vi "Delete Entity.vi"(8 "error in (no error)":errorcluster, 9 "enqueuer":refnum<class "Message Enqueuer.lvclass">, 10 "entity type":i32, 11 "entity table in":refnum<class "Entity Table.lvclass">) -> (0 "error out":errorcluster, 3 "entity table out":refnum<class "Entity Table.lvclass">)   [LabVIEW 2020, in "Entity Table.lvclass"]
doc: "Delete an actor from the entity table."
uses:
  Entity Table.lvclass
  <vilib>/ActorFramework/Message Enqueuer/Message Enqueuer.lvclass
  Entity Table.lvclass/Entity Table.ctl
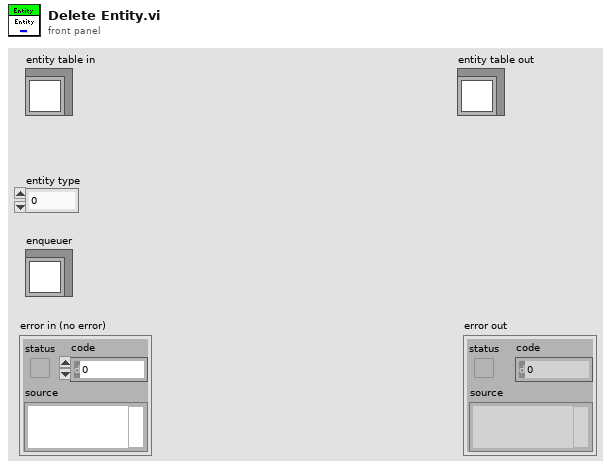
[diagram p1: front panel]
types:
  T1 = typedef "Entity Table.lvclass/Entity Table Element.ctl" = cluster{"Entity":refnum<class "Message Enqueuer.lvclass">[], "Entity Data":T2[]}
  T2 = typedef "Entity Table.lvclass/Entity Data.ctl" = cluster{"Name":string, "Status":string}
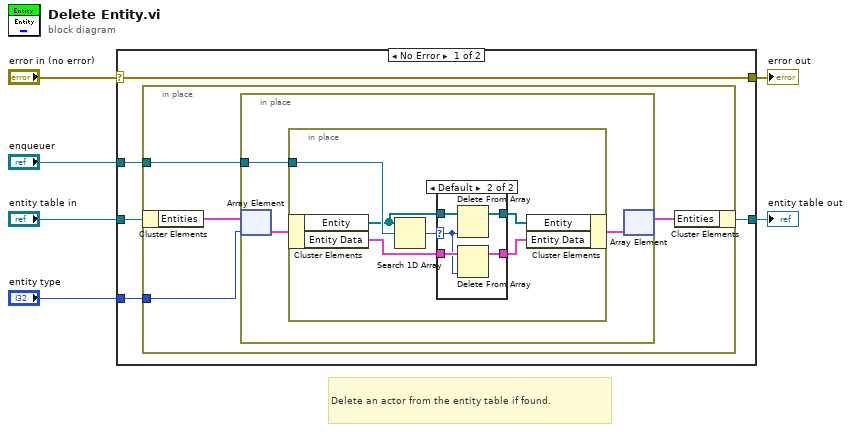
[diagram p0: block diagram]
diagram:
  # "Delete an actor from the entity table if found."
  n1 = case shown="No Error" "error in (no error)" {
    selector: "error in (no error)" -> [w9 w33]
    tunnel: [w9 w33] -> w5
    tunnel: "entity table in" -> [w8 w32]
    tunnel: [w7 w32] -> w3
    tunnel: "entity type" -> [w11 _]
    tunnel: "enqueuer" -> [w10 _]
    frame No Error {
      n2 = in-place "In Place Element Structure" {
        in-place-border: w11 -> [w15]
        in-place-border: w10 -> [w14]
        n3 = in-place-cluster #1 ("Unbundle / Bundle Elements")(w8) -> ("Entities"=w13:T1[])
        n4 = in-place "In Place Element Structure" {
          in-place-border: w14 -> [w17]
          n5 = in-place-array #2 ("Array Index / Replace Elements")(w13, w15) -> (w18:T1)
          n6 = in-place "In Place Element Structure" {
            in-place-border: w17 -> [w24]
            n7 = in-place-cluster #3 ("Unbundle / Bundle Elements")(w18) -> ("Entity"=w21:refnum<class "Message Enqueuer.lvclass">[], "Entity Data"=w20:T2[])
            n8 = Search 1D Array(1D array=w21, element=w24) -> (index of element=w23:i32)  [unwired: 1 in]
            n9 = case shown="Default" w23 {
              selector: w23 -> [_ w27]
              tunnel: [w26 w30] -> w22
              tunnel: w21 -> [w26 w31]
              tunnel: w20 -> [w25 w29]
              tunnel: [w25 w28] -> w19
              frame -1 {
              }
              frame Default {
                n10 = Delete From Array(array=w31, index=w27) -> (array with subset deleted=w30:refnum<class "Message Enqueuer.lvclass">[])  [unwired: 1 in, 1 out]
                n11 = Delete From Array(array=w29, index=w27) -> (array with subset deleted=w28:T2[])  [unwired: 1 in, 1 out]
              }
            }
            n12 = in-place-cluster #3 ("Unbundle / Bundle Elements")("Entity"=w22, "Entity Data"=w19) -> (w16:T1)
          }
          n13 = in-place-array #2 ("Array Index / Replace Elements")(w16) -> (w12:T1[])  [unwired: 1 out]
        }
        n14 = in-place-cluster #1 ("Unbundle / Bundle Elements")("Entities"=w12) -> (w7:refnum<class "Entity Table.lvclass">)
      }
    }
    frame Error {
    }
  }
  "error out" <- w5
  "entity table out" <- w3
